vi "Determine Warnings - Exercise 3-8.vi"() -> ()   [LabVIEW 2014]
panel:
  out "Warning?":bool
  out "Warning Text":string
  in  "Min Temp":dbl
  in  "Max Temp":dbl
  in  "Current Temp":dbl
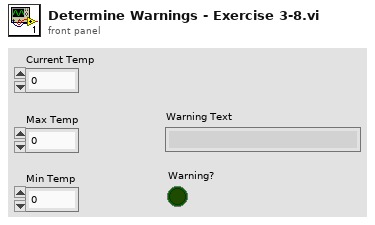
[diagram p1: front panel]
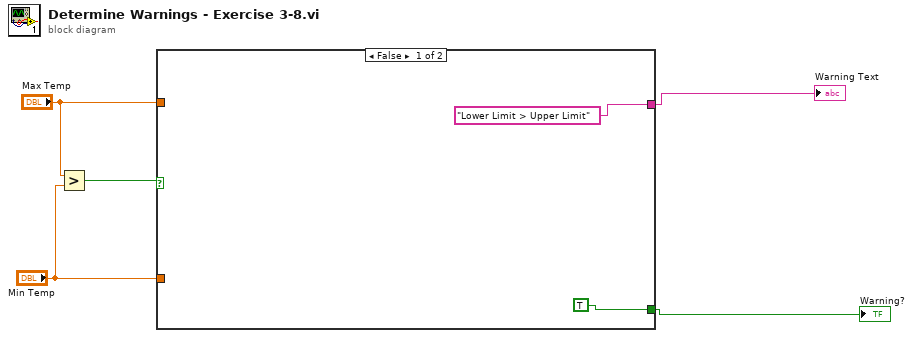
[diagram p0: block diagram]
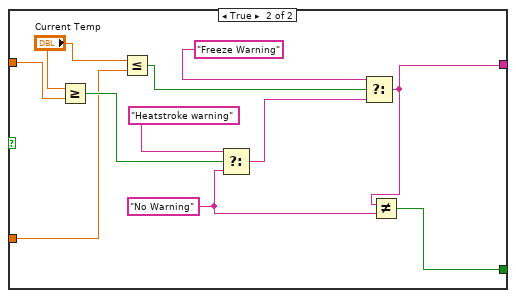
[diagram p2: hidden frame]
diagram:
  n1 = Greater?(x="Max Temp", y="Min Temp") -> (0:w3:bool)
  n2 = case shown="False" w3 {
    tunnel: ["Lower Limit > Upper Limit" w9] -> w5
    tunnel: [TRUE w13] -> w4
    tunnel: "Max Temp" -> [_ w12]
    tunnel: "Min Temp" -> [_ w10]
    frame False {
    }
    frame True {
      w14 = "No Warning"
      n3 = Greater Or Equal?(x="Current Temp", y=w12) -> (x >= y?=w18:bool)
      n4 = Less Or Equal?(x="Current Temp", y=w10) -> (x <= y?=w8:bool)
      n5 = Select(t="Heatstroke warning", s=w18, f=w14) -> (s? t:f=w16:string)
      n6 = Select(t="Freeze Warning", s=w8, f=w16) -> (s? t:f=w9:string)
      n7 = Not Equal?(x=w9, y=w14) -> (x != y?=w13:bool)
    }
  }
  "Warning Text" <- w5
  "Warning?" <- w4
